vi "ALU.vi"() -> ()   [LabVIEW 2019]
uses:
  <vilib>/Platform/TimedLoop/XDataNode/timing_clust.ctl
  <vilib>/Platform/TimedLoop/XDataNode/nitl_modes.ctl
  <vilib>/Platform/TimedLoop/XDataNode/wakeup.ctl
  <vilib>/rvi/IPIntegrationNode/IPINode_Typedef/niFpgaIPINodeSupportedFamilies.ctl
  <vilib>/rvi/IPIntegrationNode/IPINode_Utilities/niFpgaIPINodeSimCore.vi
  <vilib>/platform/TimedLoop/XDataNode/XDataNode.xnode
  <vilib>/rvi/IPIntegrationNode/IPINode_Xnode/niFpgaIPINode.xnode
  Logicas/ANDSimFiles/xsim.dir/AND/xsimkC9FA62B22FF742169113DF939251197B.dll
  Aritmeticas/SUMADORSimFiles/xsim.dir/Sumador_4/xsimk1428AA0E7BD04B74B1D6CD425682390E.dll
  Logicas/NOTSimFiles/xsim.dir/NOT/xsimk5E63DD80D0014E6EAE7248868FF032E3.dll
  Logicas/XORSimFiles/xsim.dir/XOR/xsimkCAF4F543F276499BA3178B82AF53E1F8.dll
  Logicas/ORSimFiles/xsim.dir/OR/xsimk402ADFEDA1F641FC8157E76DF9257DFC.dll
  Logicas/XOR2SimFiles/xsim.dir/XOR/xsimk3BC4A10F6C3643389904FC1C156131ED.dll
  Aritmeticas/SUMADOR_1SimFiles/xsim.dir/Sumador_4/xsimkDA9DDA9343D54E74A5744A89C1C265E9.dll
  Aritmeticas/IP_BlockSimFiles/xsim.dir/Sumador_4/xsimk2E9677DC8AC44366AD7A188DC0AF548C.dll
  Flags/NOT_2_1SimFiles/xsim.dir/Zero/xsimk50B6D53BD3D347F78EDDDD46F14DB283.dll
  Mux/MUX_8_1SimFiles/xsim.dir/Mux/xsimk3AA67113D66D4B2BBB2962C1CC624604.dll
  Logicas/NOT_2SimFiles/xsim.dir/NOT/xsimkADC4F42F1B0F426FB45CA22F1F060483.dll
  Mux/MUX_8_1_4SimFiles/xsim.dir/Mux/xsimk3C0E5E4E319C46D7BDD04E9AA4B0685F.dll
  <vilib>/Platform/TimedLoop/XDataNode/XDNodeRunTimeDep.lvlib
panel:
  in  "Tab Control":enum32{"Page 1"}(tab)
  in  "S_2":bool
  in  "S_1":bool
  in  "S_0":bool
  in  "INA1":bool
  in  "INA2":bool
  in  "INA3":bool
  in  "INA4":bool
  in  "INB1":bool
  in  "INB2":bool
  in  "INB3":bool
  in  "INB4":bool
  out "?":T1
  out "Zero":bool
  out "XOR":T2
  out "NOT A":T2
  out "Suma":T2
  out "Resta":T2
  out "AND":T2
  out "OR":T2
  out "Multiplicador":T3
  out "Cout":bool
  # "Funciones"
  # "Operaciones"
  # "S2   S1   S0    F\n0      0     0     A+B\n0      0     1     A-B\n0      1     0     A*B\n0      1     1     --\n1      0     0     A and B\n1      0     1     A  or   B\n1      1     0     A  xor B\n1      1     1     not A"
  # "Selección"
  # "A"
  # "B"
  # "Salida"
  # "Banderas"
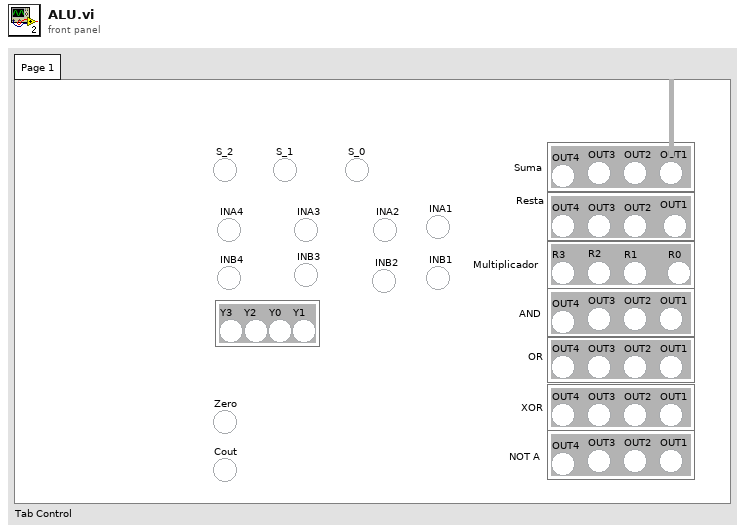
[diagram p1: front panel]
types:
  T1 = cluster{"Y3":bool, "Y2":bool, "Y0":bool, "Y1":bool}
  T2 = cluster{"OUT1":bool, "OUT2":bool, "OUT3":bool, "OUT4":bool}
  T3 = cluster{"R0":bool, "R1":bool, "R2":bool, "R3":bool}
  T4 = typedef "XDNodeRunTimeDep.lvlib/timing_clust.ctl" = cluster{"Expected End [f-1]":u64, "Actual End [f-1]":u64, "Finished Late? [f-1]":bool, "Expected End [i-1]":u64, "Actual End [i-1]":u64, "Finished Late? [i-1]":bool, "Expected Start [i]":u64, "Actual Start [i]":u64, "Expected Start [f]":u64, "Actual Start [f]":u64, "Source Name":string, "Structure Name":string, "Period":i64, "Deadline":i64, "Offset":i64, "Start":i64, "Priority":i32, "Timeout":i32, "Mode":T5, "Wakeup Reason":T6, "Error":errorcluster, "Source Type":string, "Secondary Source Type":string, "Global End Time":u64, "Global Start Time":u64, "Frame Duration":u64, "Iteration Duration":u64, "Assigned CPU":i32, "I/O Scan Engine Mode":u32}
  T5 = typedef "XDNodeRunTimeDep.lvlib/nitl_modes.ctl" = enum32{"No Change", "Process missed periods, maintain original phase", "Discard missed periods, maintain original phase", "Process missed periods, ignore original phase", "Discard missed periods, ignore original phase"}
  T6 = typedef "XDNodeRunTimeDep.lvlib/wakeup.ctl" = enum32{"Normal", "Aborted", "Asynchronous wakeup", "Timing source error", "Timed loop error", "Timeout"}
  T7 = typedef "niFpgaIPINodeSupportedFamilies.ctl" = cluster{"unlimited?":bool, "supported targets":string[]}
  T8 = cluster{"INA1":bool, "INA2":bool, "INA3":bool, "INA4":bool, "INB1":bool, "INB2":bool, "INB3":bool, "INB4":bool}
  T9 = cluster{"O1":bool, "O2":bool, "O3":bool, "O4":bool}
  T10 = cluster{"Y3":bool, "Y2":bool, "Y1":bool, "Y0":bool}
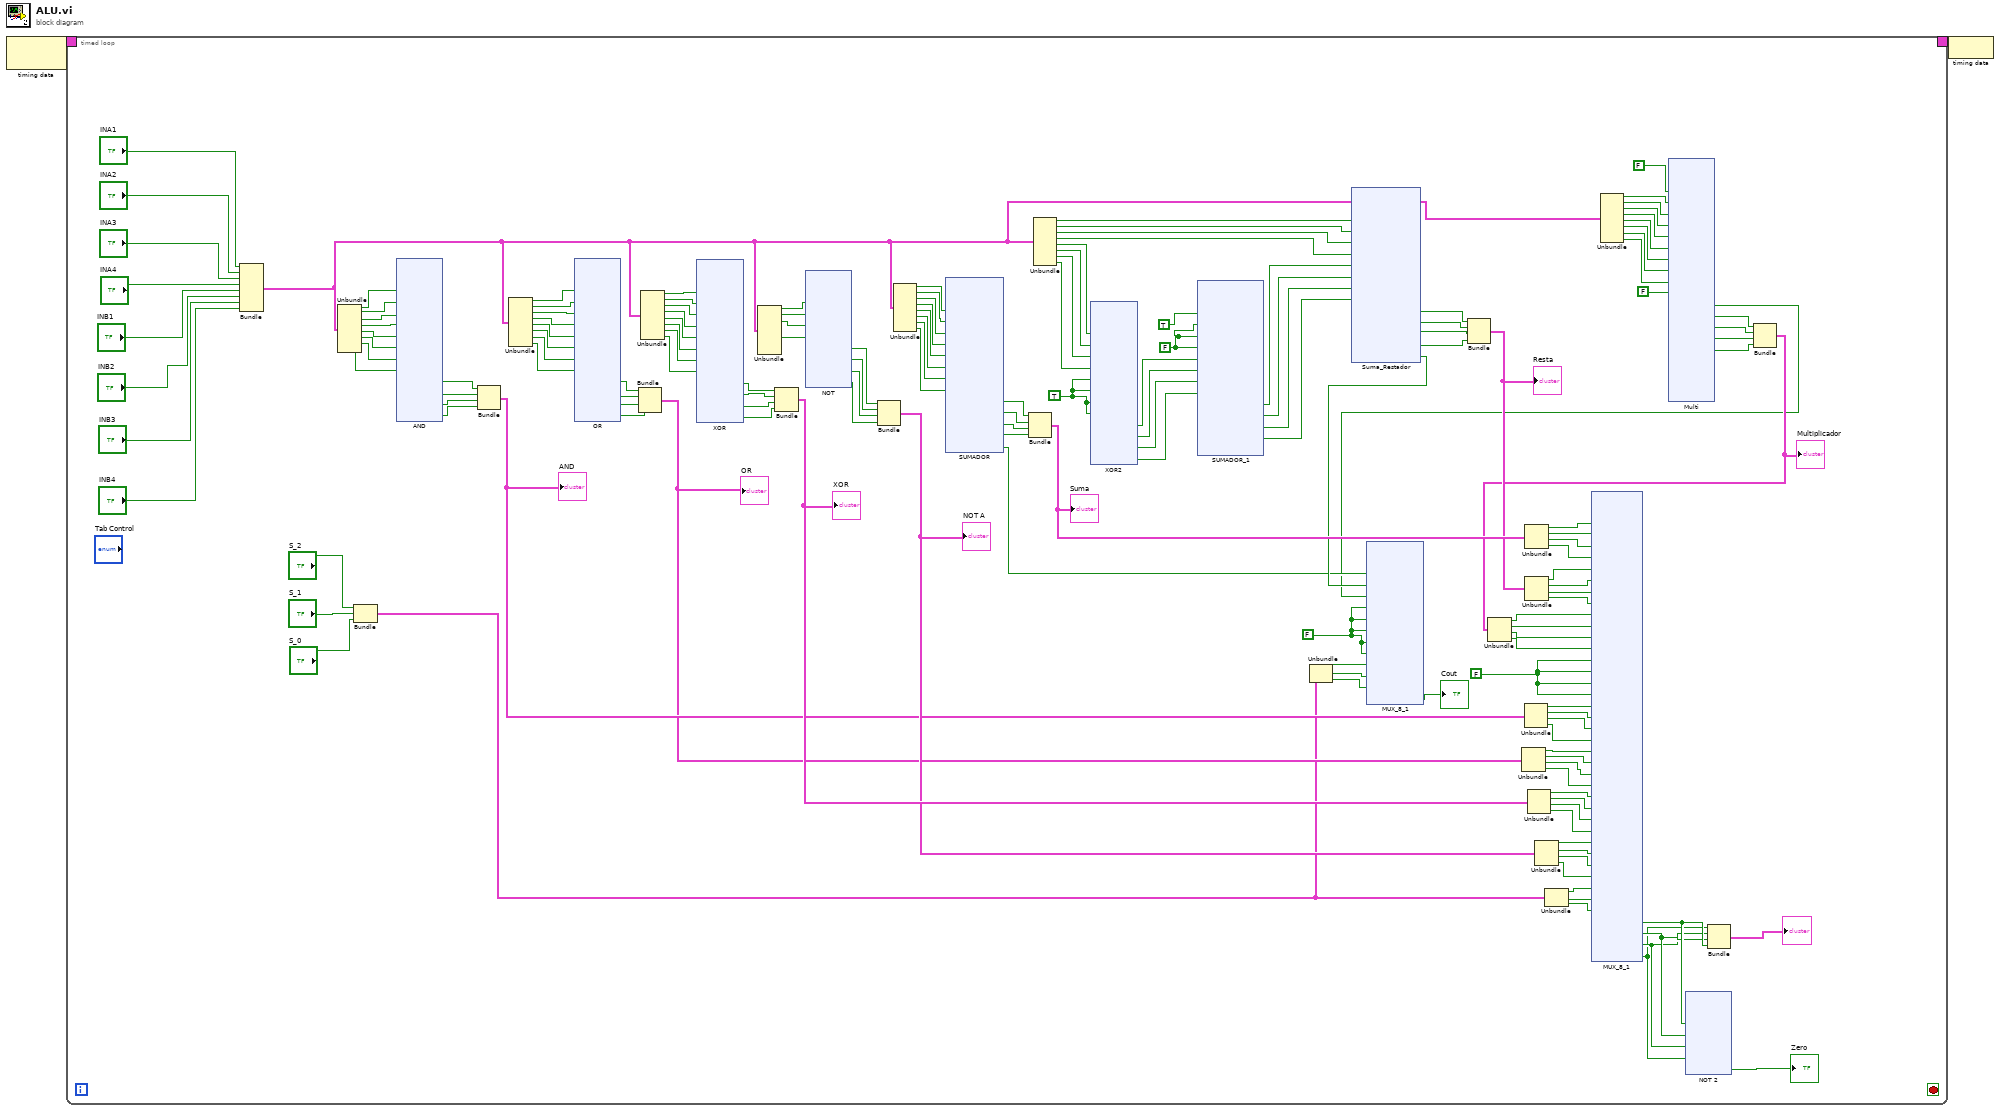
[diagram p0: block diagram]
diagram:
  n1 = node-c288() -> (w2:T4)  [unwired: 1 in]
  n2 = timed-loop {
    timing: w2 -> [_]
    timing-out: [_] -> w1
    stop <- _ stop-if-true
    w4 = FALSE ("IN3")
    w95 = FALSE ("IN02")
    w62 = FALSE ("A3")
    w138 = TRUE ("INB1")
    n3 = Bundle("INA1"="INA1", "INA2"="INA2", "INA3"="INA3", "INA4"="INA4", "INB1"="INB1", "INB2"="INB2", "INB3"="INB3", "INB4"="INB4") -> (w54:T8)  [unwired: 1 in]
    n4 = Unbundle(w54) -> ("INA1"=w157:bool, "INA2"=w156:bool, "INA3"=w155:bool, "INA4"=w154:bool, "INB1"=w40:bool, "INB2"=w39:bool, "INB3"=w38:bool, "INB4"=w37:bool)
    n5 = Bundle("S_2"="S_2", "S_1"="S_1", "S_0"="S_0") -> (w5:cluster{"S_2":bool, "S_1":bool, "S_0":bool})  [unwired: 1 in]
    n6 = xnode ("AND")("INA1"=w157, "INA2"=w156, "INA3"=w155, "INA4"=w154, "INB1"=w40, "INB2"=w39, "INB3"=w38, "INB4"=w37) -> ("OUT1"=w114:bool, "OUT2"=w115:bool, "OUT3"=w116:bool, "OUT4"=w117:bool)
    n7 = Bundle("OUT1"=w114, "OUT2"=w115, "OUT3"=w116, "OUT4"=w117) -> (w73:T2)  [unwired: 1 in]
    "AND" <- w73
    n8 = Unbundle(w54) -> ("INA1"=w153:bool, "INA2"=w152:bool, "INA3"=w151:bool, "INA4"=w150:bool, "INB1"=w23:bool, "INB2"=w22:bool, "INB3"=w21:bool, "INB4"=w20:bool)
    n9 = xnode ("OR")("INA1"=w153, "INA2"=w152, "INA3"=w151, "INA4"=w150, "INB1"=w23, "INB2"=w22, "INB3"=w21, "INB4"=w20) -> ("OUT1"=w133:bool, "OUT2"=w132:bool, "OUT3"=w131:bool, "OUT4"=w130:bool)
    n10 = Bundle("OUT1"=w133, "OUT2"=w132, "OUT3"=w131, "OUT4"=w130) -> (w72:T2)  [unwired: 1 in]
    "OR" <- w72
    n11 = Unbundle(w54) -> ("INA1"=w149:bool, "INA2"=w148:bool, "INA3"=w147:bool, "INA4"=w146:bool, "INB1"=w27:bool, "INB2"=w26:bool, "INB3"=w25:bool, "INB4"=w24:bool)
    n12 = xnode ("XOR")("INA1"=w149, "INA2"=w148, "INA3"=w147, "INA4"=w146, "INB1"=w27, "INB2"=w26, "INB3"=w25, "INB4"=w24) -> ("OUT1"=w129:bool, "OUT2"=w128:bool, "OUT3"=w127:bool, "OUT4"=w126:bool)
    n13 = Unbundle(w54) -> ("INA1"=w145:bool, "INA2"=w144:bool, "INA3"=w143:bool, "INA4"=w142:bool)  [unwired: 4 out]
    n14 = Bundle("OUT1"=w129, "OUT2"=w128, "OUT3"=w127, "OUT4"=w126) -> (w77:T2)  [unwired: 1 in]
    "XOR" <- w77
    n15 = xnode ("NOT")("INA1"=w145, "INA2"=w144, "INA3"=w143, "INA4"=w142) -> ("OUT1"=w125:bool, "OUT2"=w124:bool, "OUT3"=w123:bool, "OUT4"=w122:bool)
    n16 = Bundle("OUT1"=w125, "OUT2"=w124, "OUT3"=w123, "OUT4"=w122) -> (w76:T2)  [unwired: 1 in]
    "NOT A" <- w76
    n17 = Unbundle(w54) -> ("INA1"=w141:bool, "INA2"=w140:bool, "INA3"=w139:bool, "INA4"=w33:bool, "INB1"=w31:bool, "INB2"=w30:bool, "INB3"=w29:bool, "INB4"=w28:bool)
    n18 = xnode ("SUMADOR")("A0"=w141, "A1"=w140, "A2"=w139, "A3"=w33, "B0"=w31, "B1"=w30, "B2"=w29, "B3"=w28) -> ("O1"=w121:bool, "O2"=w120:bool, "O3"=w118:bool, "O4"=w119:bool, "Cout"=w10:bool)
    n19 = Bundle("O1"=w121, "O2"=w120, "O3"=w118, "O4"=w119) -> (w75:T9)  [unwired: 1 in]
    "Suma" <- w75
    n20 = Unbundle(w54) -> ("INA1"=w137:bool, "INA2"=w136:bool, "INA3"=w135:bool, "INA4"=w134:bool, "INB1"=w36:bool, "INB2"=w35:bool, "INB3"=w34:bool, "INB4"=w32:bool)
    n21 = xnode ("XOR2")("INA1"=w36, "INA2"=w35, "INA3"=w34, "INA4"=w32, "INB1"=w138, "INB2"=w138, "INB3"=w138, "INB4"=w138) -> ("OUT1"=w67:bool, "OUT2"=w66:bool, "OUT3"=w64:bool, "OUT4"=w65:bool)
    n22 = xnode ("SUMADOR_1")("A0"=TRUE ("A3"), "A1"=w62, "A2"=w62, "A3"=w62, "B0"=w67, "B1"=w66, "B2"=w64, "B3"=w65) -> ("O1"=w71:bool, "O2"=w70:bool, "O3"=w69:bool, "O4"=w68:bool)  [unwired: 1 out]
    n23 = Unbundle(w5) -> ("S_2"=w8:bool, "S_1"=w7:bool, "S_0"=w6:bool)
    n24 = xnode ("Suma_Restador")("A0"=w137, "A1"=w136, "A2"=w135, "A3"=w134, "B0"=w71, "B1"=w70, "B2"=w69, "B3"=w68) -> ("O1"=w99:bool, "O2"=w98:bool, "O3"=w97:bool, "O4"=w96:bool, "Cout"=w11:bool)
    n25 = Bundle("O1"=w99, "O2"=w98, "O3"=w97, "O4"=w96) -> (w74:T9)  [unwired: 1 in]
    "Resta" <- w74
    n26 = Unbundle(w72) -> ("OUT1"=w90:bool, "OUT2"=w89:bool, "OUT3"=w87:bool, "OUT4"=w88:bool)
    n27 = Unbundle(w73) -> ("OUT1"=w94:bool, "OUT2"=w93:bool, "OUT3"=w92:bool, "OUT4"=w91:bool)
    n28 = Unbundle(w75) -> ("O1"=w107:bool, "O2"=w106:bool, "O3"=w105:bool, "O4"=w104:bool)
    n29 = Unbundle(w74) -> ("O1"=w103:bool, "O2"=w102:bool, "O3"=w101:bool, "O4"=w100:bool)
    n30 = Unbundle(w77) -> ("OUT1"=w86:bool, "OUT2"=w85:bool, "OUT3"=w84:bool, "OUT4"=w83:bool)
    n31 = Unbundle(w76) -> ("OUT1"=w79:bool, "OUT2"=w80:bool, "OUT3"=w81:bool, "OUT4"=w82:bool)
    n32 = Unbundle(w5) -> ("S_2"=w110:bool, "S_1"=w109:bool, "S_0"=w108:bool)
    n33 = Unbundle(w54) -> ("INA1"=w19:bool, "INA2"=w18:bool, "INA3"=w17:bool, "INA4"=w16:bool, "INB1"=w15:bool, "INB2"=w14:bool, "INB3"=w13:bool, "INB4"=w12:bool)
    n34 = xnode ("Multi")("ZeroI"=FALSE, "A0"=w19, "A1"=w18, "A2"=w17, "A3"=w16, "B0"=w15, "B1"=w14, "B2"=w13, "B3"=w12, "Cin"=FALSE) -> ("Cout"=w9:bool, "R0"=w53:bool, "R1"=w52:bool, "R2"=w51:bool, "R3"=w50:bool)  [unwired: 4 out]
    n35 = xnode ("MUX_8_1")("IN0"=w10, "IN1"=w11, "IN2"=w9, "IN3"=w4, "IN4"=w4, "IN5"=w4, "IN6"=w4, "IN7"=w4, "S0"=w8, "S1"=w7, "S2"=w6) -> ("Y"=→"Cout":bool)
    n36 = Bundle("R0"=w53, "R1"=w52, "R2"=w51, "R3"=w50) -> (w49:T3)  [unwired: 1 in]
    "Multiplicador" <- w49
    n37 = Unbundle(w49) -> ("R0"=w48:bool, "R1"=w47:bool, "R2"=w46:bool, "R3"=w45:bool)
    n38 = xnode ("MUX_8_1")("IN00"=w107, "IN10"=w106, "IN20"=w105, "IN30"=w104, "IN01"=w103, "IN11"=w102, "IN21"=w101, "IN31"=w100, "IN02"=w48, "IN12"=w47, "IN22"=w46, "IN32"=w45, "IN03"=w95, "IN13"=w95, "IN23"=w95, "IN33"=w95, "IN04"=w94, "IN14"=w93, "IN24"=w92, "IN34"=w91, "IN05"=w90, "IN15"=w89, "IN25"=w87, "IN35"=w88, "IN06"=w86, "IN16"=w85, "IN26"=w84, "IN36"=w83, "IN07"=w79, "IN17"=w80, "IN27"=w81, "IN37"=w82, "S0"=w110, "S1"=w109, "S2"=w108) -> ("Y0"=w61:bool, "Y1"=w60:bool, "Y2"=w59:bool, "Y3"=w58:bool)
    n39 = xnode ("NOT 2")("INA1"=w61, "INA2"=w60, "INA3"=w59, "INA4"=w58) -> ("OUTZ"=→"Zero":bool)
    n40 = Bundle("Y3"=w58, "Y2"=w59, "Y1"=w60, "Y0"=w61) -> (→"?":T10)  [unwired: 1 in]
  }
  n41 = node-c288(w1) -> ()
